vi "Toggle Switch Variable.vi"() -> ()   [LabVIEW 2019]
panel:
  in  "Trigger/Bumper Boolean":bool
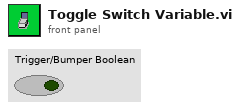
[diagram p1: front panel]
diagram:
